vi "Class - ResultCntr.TEST.vi"() -> ()   [LabVIEW 2016]
uses:
  Class - ResultCntr.lvclass
panel:
  in  "Init":bool
  in  "Result":bool
  in  "SubSection - End":bool
  in  "SubSection - Start":bool
  in  "Section - End":bool
  in  "Section - Start":bool
  out "Results":string[][](array[string])
  # "Desc"
  # "ID"
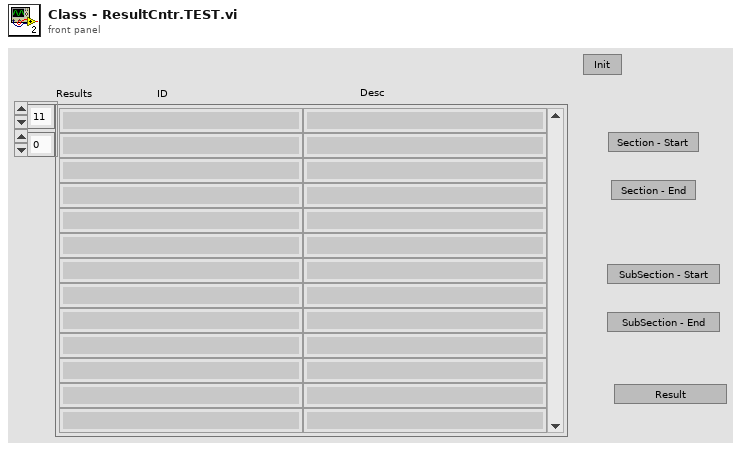
[diagram p1: front panel]
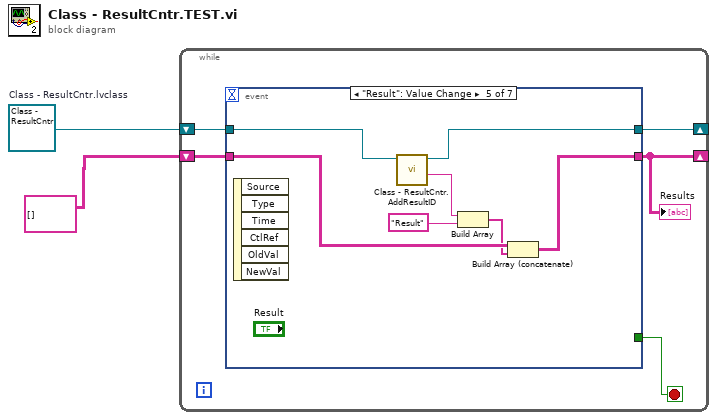
[diagram p0: block diagram]
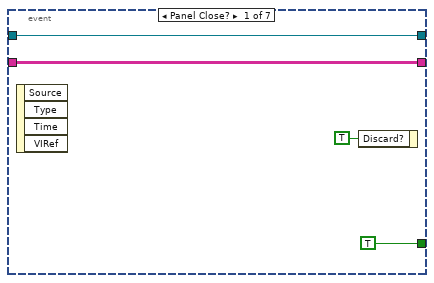
[diagram p2: hidden frame]
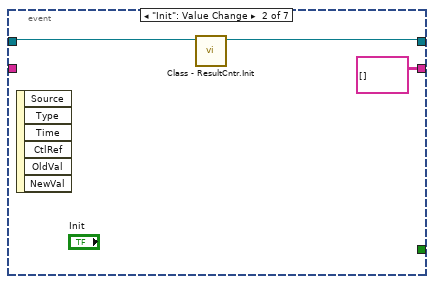
[diagram p3: hidden frame]
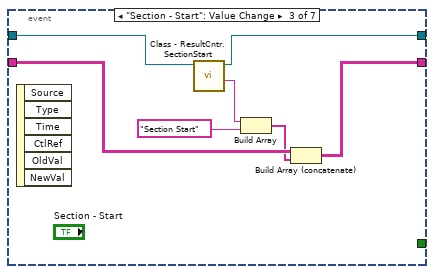
[diagram p4: hidden frame]
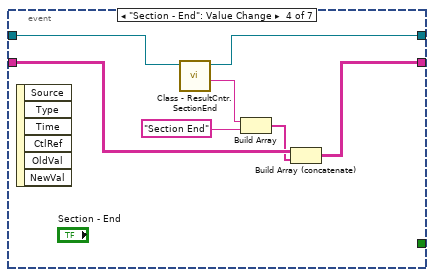
[diagram p5: hidden frame]
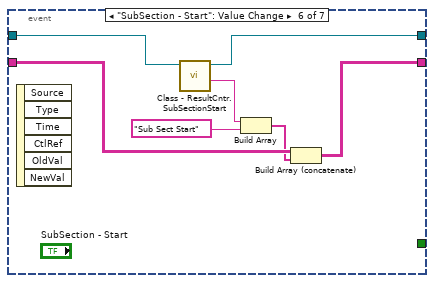
[diagram p6: hidden frame]
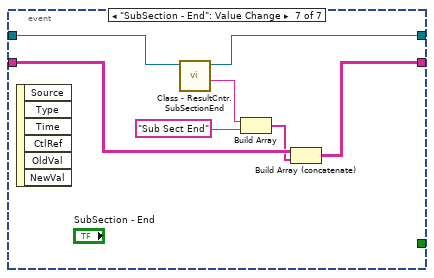
[diagram p7: hidden frame]
diagram:
  w2 = refnum<class "Class - ResultCntr.lvclass"> refnum  # Class - ResultCntr.lvclass
  n1 = while {
    shift-right: [w5] -> _
    shift-left: w2 -> [w7]
    shift-right: [w3] -> _
    shift-left: string[][] [] -> [w6]
    stop <- w4 stop-if-true
    n2 = event shown="[4] \"Result\": Value Change" {
      selector: _ -> [_ _ _ _ _ _ _]
      dyn-events: _ -> [_ _ _ _ _ _ _]
      timeout: _ -> [_ _ _ _ _ _ _]
      tunnel: w7 -> [w10 w13 w21 w28 w35 w42 w49]
      tunnel: w6 -> [w11 _ w19 w26 w33 w40 w47]
      tunnel: [w11 string[][] [] w15 w22 w29 w36 w43] -> w3
      tunnel: [w10 w12 w20 w27 w34 w41 w48] -> w5
      tunnel: [TRUE ("Discard?") _ _ _ _ _ _] -> w4
      event Panel Close? {
        n3 = event-data() -> ()  [unwired: 1 in, 4 out]
        n4 = event-data("Discard?"=TRUE) -> ()  [unwired: 1 in, 1 out]
      }
      event "Init": Value Change {
        n5 = event-data() -> ()  [unwired: 1 in, 6 out]
        n6 = call "Class - ResultCntr.Init.vi"("Class - ResultCntr in"=w13) -> ("Class - ResultCntr out"=w12:refnum<class "Class - ResultCntr.lvclass">)  [unwired: 9 in, 1 out]
      }
      event "Section - Start": Value Change {
        n7 = event-data() -> ()  [unwired: 1 in, 6 out]
        n8 = call "Class - ResultCntr.SectionStart.vi"("Class - ResultCntr in"=w21) -> ("ID"=w18:string, "Class - ResultCntr out"=w20:refnum<class "Class - ResultCntr.lvclass">)  [unwired: 8 in, 1 out]
        n9 = Build Array(w18, "Section Start" ("element")) -> (w16:string[])
        n10 = Build Array (concatenate)(w19, w16) -> (w15:string[][])
      }
      event "Section - End": Value Change {
        n11 = event-data() -> ()  [unwired: 1 in, 6 out]
        n12 = call "Class - ResultCntr.SectionEnd.vi"("Class - ResultCntr in"=w28) -> ("ID"=w25:string, "Class - ResultCntr out"=w27:refnum<class "Class - ResultCntr.lvclass">)  [unwired: 8 in, 1 out]
        n13 = Build Array(w25, "Section End" ("element")) -> (w23:string[])
        n14 = Build Array (concatenate)(w26, w23) -> (w22:string[][])
      }
      event "Result": Value Change {
        n15 = event-data() -> ()  [unwired: 1 in, 6 out]
        n16 = call "Class - ResultCntr.AddResultID.vi"("Class - ResultCntr in"=w35) -> ("ID"=w32:string, "Class - ResultCntr out"=w34:refnum<class "Class - ResultCntr.lvclass">)  [unwired: 8 in, 1 out]
        n17 = Build Array(w32, "Result" ("element")) -> (w30:string[])
        n18 = Build Array (concatenate)(w33, w30) -> (w29:string[][])
      }
      event "SubSection - Start": Value Change {
        n19 = event-data() -> ()  [unwired: 1 in, 6 out]
        n20 = call "Class - ResultCntr.SubSectionStart.vi"("Class - ResultCntr in"=w42) -> ("ID"=w39:string, "Class - ResultCntr out"=w41:refnum<class "Class - ResultCntr.lvclass">)  [unwired: 8 in, 1 out]
        n21 = Build Array(w39, "Sub Sect Start" ("element")) -> (w37:string[])
        n22 = Build Array (concatenate)(w40, w37) -> (w36:string[][])
      }
      event "SubSection - End": Value Change {
        n23 = event-data() -> ()  [unwired: 1 in, 6 out]
        n24 = call "Class - ResultCntr.SubSectionEnd.vi"("Class - ResultCntr in"=w49) -> ("ID"=w46:string, "Class - ResultCntr out"=w48:refnum<class "Class - ResultCntr.lvclass">)  [unwired: 8 in, 1 out]
        n25 = Build Array(w46, "Sub Sect End" ("element")) -> (w44:string[])
        n26 = Build Array (concatenate)(w47, w44) -> (w43:string[][])
      }
    }
    "Results" <- w3
  }
